vi "CH_LM Action Configuration Delete.vi"(0 "Meter Index":i32, 2 "Configuration File Name (\"\")":string, 5 "error in (no error)":errorcluster, 7 "Timeout / ms (3000)":i32=3000, 9 "Lock Timeout / ms (1000)":i32=1000) -> (11 "Lock timed out":bool, 14 "Meter Index":i32, 19 "error out":errorcluster)   [LabVIEW 2012, in "CH_LM.lvlib"]
doc: "This command will delete the named configuration file.\n\n<B>Attention:</B> An attempt to delete a non-existent configuration will raise error 101. An attempt to delete the \"Factory Settings\" configuration will raise error 101."
uses:
  CH_LM.lvlib
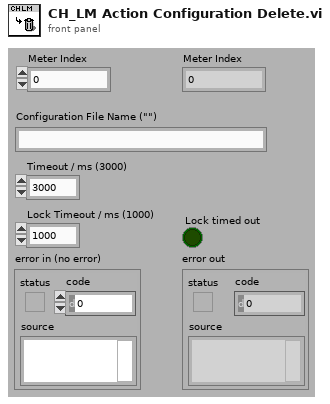
[diagram p1: front panel]
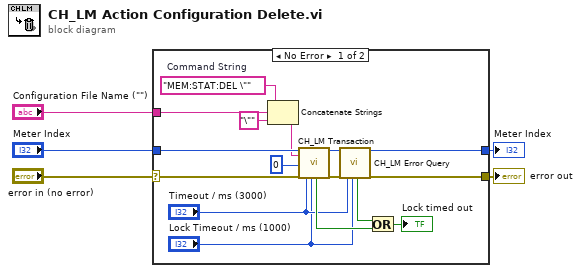
[diagram p0: block diagram]
diagram:
  n1 = case shown="No Error" "error in (no error)" {
    selector: "error in (no error)" -> [w21 w23]
    tunnel: [w18 w23] -> w5
    tunnel: "Meter Index" -> [w20 w22]
    tunnel: [w19 w22] -> w2
    tunnel: "Configuration File Name (\"\")" -> [w17 _]
    frame No Error {
      w8 = "MEM:STAT:DEL \""  # Command String
      n2 = Concatenate Strings(w8, w17, "\"" ("string")) -> (w7:string)
      n3 = call "CH_LM Transaction.vi"("Meter Index"=w20, "Command String"=w7, "NofStrings (-1:all)"=0 ("t"), "error in (no error)"=w21, "Timeout / ms (3000)"="Timeout / ms (3000)", "Lock Timeout / ms (1000)"="Lock Timeout / ms (1000)") -> ("Lock timed out"=w12:bool, "Meter Index"=w15:i32, "error out"=w14:errorcluster)  [unwired: 11 out]
      n4 = call "CH_LM Error Query.vi"("Meter Index"=w15, "error in (no error)"=w14, "Timeout / ms (3000)"="Timeout / ms (3000)", "Lock Timeout / ms (1000)"="Lock Timeout / ms (1000)") -> ("Lock timed out"=w13:bool, "Meter Index"=w19:i32, "error out"=w18:errorcluster)  [unwired: 13 out]
      n5 = Or(x=w13, y=w12) -> (x .or. y?=→"Lock timed out":bool)
    }
    frame Error {
    }
  }
  "error out" <- w5
  "Meter Index" <- w2
